vi "End of actuater limiter.vi"(9 "Lower limit switch":T1={"DevStatus"={"status"=FALSE, "code"=0, "source"=""}, "DIO Channel"=enum."DIO 1", "Controller"=enum."Controller 1", "CntIndex"=enum."Invalid", "Normally Closed"=FALSE}, 10 "Upper limit switch":T1={"DevStatus"={"status"=FALSE, "code"=0, "source"=""}, "DIO Channel"=enum."DIO 1", "Controller"=enum."Controller 1", "CntIndex"=enum."Invalid", "Normally Closed"=FALSE}, 11 "Motor input":dbl format="%#_13g") -> (3 "Motor output":dbl format="%#_13g")   [LabVIEW 2014]
uses:
  <vilib>/Rock Robotics/WPI/Switch/WPI_SwitchDevRef.ctl
  <vilib>/Rock Robotics/SystemInterfaces/DIO/FPGA_DIOChannel.ctl
  <vilib>/Rock Robotics/SystemInterfaces/Typedef/FPGA_TypedefDigitalModule.ctl
  <vilib>/Rock Robotics/SystemInterfaces/Counter/FPGA_CounterCtrSystemIndex.ctl
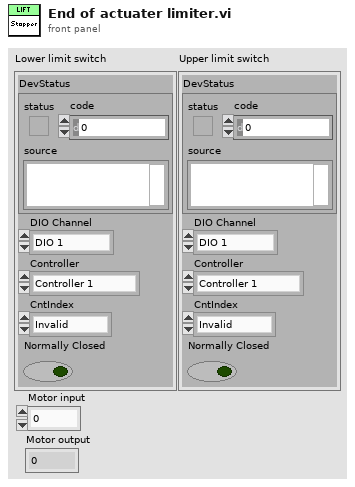
[diagram p1: front panel]
types:
  T1 = typedef "WPI_SwitchDevRef.ctl" = cluster{"DevStatus":errorcluster, "DIO Channel":T2, "Controller":T3, "CntIndex":T4, "Normally Closed":bool}
  T2 = typedef "FPGA_DIOChannel.ctl" = enum8{"DIO 0", "DIO 1", "DIO 2", "DIO 3", "DIO 4", "DIO 5", "DIO 6", "DIO 7", "DIO 8", "DIO 9", "DIO MXP 0", "DIO MXP 1", "DIO MXP 2", "DIO MXP 3", "DIO MXP 4", "DIO MXP 5", "DIO MXP 6", "DIO MXP 7", "DIO MXP 8", "DIO MXP 9", "DIO MXP 10", "DIO MXP 11", "DIO MXP 12", "DIO MXP 13", "DIO MXP 14", "DIO MXP 15", "Invalid"}
  T3 = typedef "FPGA_TypedefDigitalModule.ctl" = enum16{"Controller 1"}
  T4 = typedef "FPGA_CounterCtrSystemIndex.ctl" = enum8{"Ctr 0", "Ctr 1", "Ctr 2", "Ctr 3", "Ctr 4", "Ctr 5", "Ctr 6", "Ctr 7", "Invalid"}
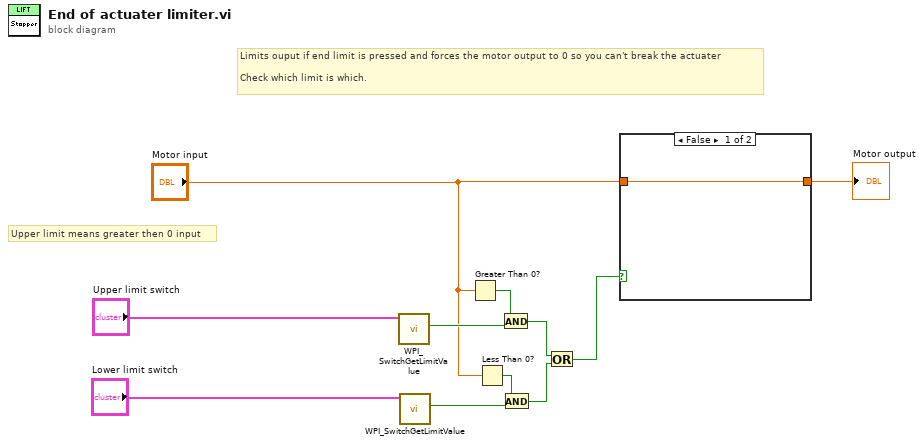
[diagram p0: block diagram]
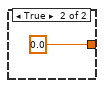
[diagram p2: hidden frame]
diagram:
  # "Limits ouput if end limit is pressed and forces the motor output to 0 so you can't break the actuater\n\nCheck which limit is which."
  # "Upper limit means greater then 0 input"
  n1 = call <vilib>:"WPI_SwitchGetLimitValue.vi"("SwitchDevRef"="Upper limit switch") -> ("Switch Pressed"=w8:bool)  [unwired: 8 in, 2 out]
  n2 = call <vilib>:"WPI_SwitchGetLimitValue.vi"("SwitchDevRef"="Lower limit switch") -> ("Switch Pressed"=w7:bool)  [unwired: 8 in, 2 out]
  n3 = Greater Than 0?(x="Motor input") -> (x > 0?=w9:bool)
  n4 = Less Than 0?(x="Motor input") -> (x < 0?=w6:bool)
  n5 = And(x=w9, y=w8) -> (x .and. y?=w5:bool)
  n6 = And(x=w6, y=w7) -> (x .and. y?=w4:bool)
  n7 = Or(x=w5, y=w4) -> (x .or. y?=w3:bool)
  n8 = case shown="False" w3 {
    tunnel: "Motor input" -> [w12 _]
    tunnel: [w12 0.0 ("Motor input")] -> w1
    frame False {
    }
    frame True {
    }
  }
  "Motor output" <- w1
